vi "chr63204A_Load_State.vi"(8 "error in (no error)":errorcluster, 10 "LOAD":bool, 11 "VISA resource name":refnum<visa-resource-name>) -> (0 "error out":errorcluster, 3 "VISA resource name out":refnum<visa-resource-name>)   [LabVIEW 2020]
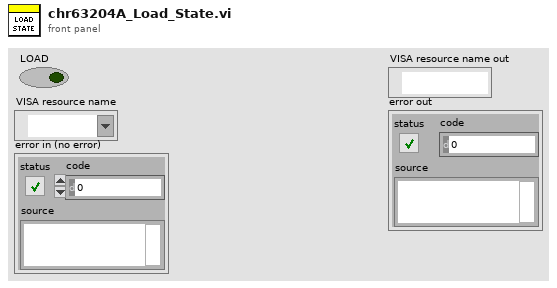
[diagram p1: front panel]
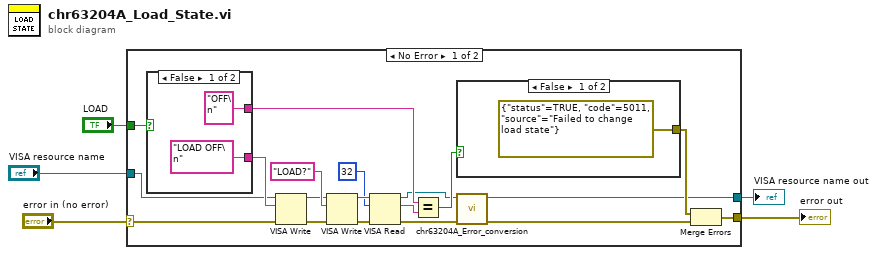
[diagram p0: block diagram]
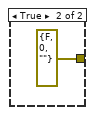
[diagram p2: hidden frame]
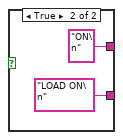
[diagram p3: hidden frame]
diagram:
  n1 = case shown="No Error" "error in (no error)" {
    selector: "error in (no error)" -> [w21 w31]
    tunnel: "LOAD" -> [w24 _]
    tunnel: "VISA resource name" -> [w22 w32]
    tunnel: [w6 w32] -> w2
    tunnel: [w11 w31] -> w1
    frame No Error {
      n2 = case shown="False" w24 {
        tunnel: ["LOAD OFF\n" "LOAD ON\n"] -> w23
        tunnel: ["OFF\n" "ON\n"] -> w13
        frame False {
        }
        frame True {
        }
      }
      n3 = VISA Write(VISA resource name=w22, write buffer=w23, error in (no error)=w21) -> (VISA resource name out=w19:refnum<visa-resource-name>, error out=w16:errorcluster)  [unwired: 1 out]
      n4 = VISA Write(VISA resource name=w19, write buffer="LOAD?", error in (no error)=w16) -> (VISA resource name out=w18:refnum<visa-resource-name>, error out=w17:errorcluster)  [unwired: 1 out]
      n5 = VISA Read(VISA resource name=w18, byte count=u32 32, error in (no error)=w17) -> (VISA resource name out=w9:refnum<visa-resource-name>, read buffer=w14:string, error out=w8:errorcluster)  [unwired: 1 out]
      n6 = Equal?(x=w13, y=w14) -> (x = y?=w12:bool)
      n7 = case shown="False" w12 {
        tunnel: [errorcluster {"status"=TRUE, "code"=5011, "source"="Failed to change load state"} ("error constant") errorcluster {"status"=FALSE, "code"=0, "source"=""} ("error constant")] -> w10
        frame False {
        }
        frame True {
        }
      }
      n8 = call "chr63204A_Error_conversion.vi"("error in (no error)"=w8, "VISA resource name"=w9) -> ("error out"=w7:errorcluster, "VISA resource name out"=w6:refnum<visa-resource-name>)  [unwired: 8 in]
      n9 = Merge Errors(w10, w7) -> (w11:errorcluster)
    }
    frame Error {
    }
  }
  "VISA resource name out" <- w2
  "error out" <- w1
